vi "Active Line Name.vi"(8 "error in":errorcluster, 11 "Multi Column Listbox in":refnum<class "Multi Column Listbox.lvclass">) -> (0 "error out":errorcluster, 2 "Active Line Name":string, 3 "Multi Column Listbox out":refnum<class "Multi Column Listbox.lvclass">)   [LabVIEW 2013, in "Table Manager.lvlib" / "Multi Column Listbox.lvclass"]
uses:
  Multi Column Listbox.lvclass
  Multi Column Listbox.lvclass/Multi Column Listbox.ctl
panel:
  in  "tag select":i32(listbox)=1
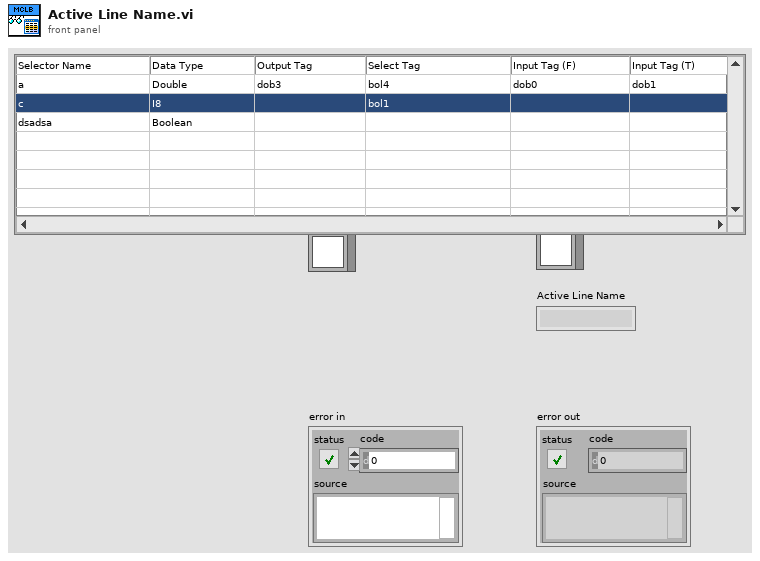
[diagram p1: front panel]
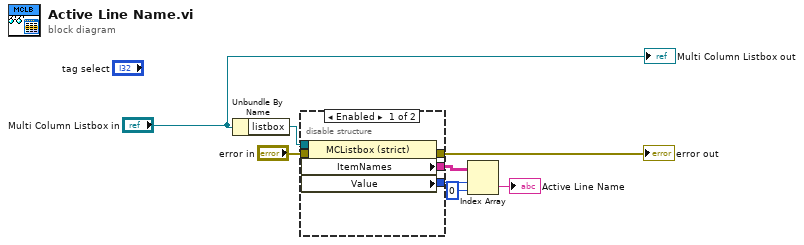
[diagram p0: block diagram]
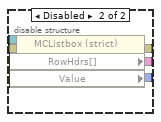
[diagram p2: hidden frame]
diagram:
  n1 = Unbundle By Name("Multi Column Listbox in") -> ("listbox"=w6:refnum<vi>)
  n2 = disable-structure shown="Enabled" {
    disable-tunnel: [w13 w18] -> w8
    disable-tunnel: [w12 w17] -> w7
    disable-tunnel: w6 -> [w11 w16]
    disable-tunnel: "error in" -> [w10 w15]
    disable-tunnel: [w9 w14] -> w2
    frame Enabled {
      n3 = property class="MCListbox (strict)"(reference=w11, error in=w10) -> (error out=w9:errorcluster, "ItemNames"=w13:string[][], "Value"=w12:i32)  [unwired: 1 out]
    }
    frame Disabled {
      n4 = property class="MCListbox (strict)"(reference=w16, error in=w15) -> (error out=w14:errorcluster, "RowHdrs[]"=w18:string[], "Value"=w17:i32)  [unwired: 1 out]
    }
  }
  "error out" <- w2
  n5 = Index Array(array=w8, index (row)=w7, index (col)=0 ("disabled index (col)")) -> (element=→"Active Line Name":string)
  "Multi Column Listbox out" <- "Multi Column Listbox in"
